vi "Msg Listened To.vi"(7 "Actor in":refnum<class "Actor.lvclass">) -> (2 "Msg Listened To":bool)   [LabVIEW 2020, in "jettl.lvlib"]
uses:
  jettl.lvlib
  Actor/Actor.lvclass
  Msg/Msg.lvclass
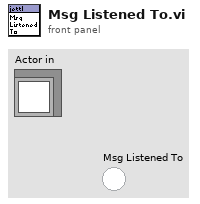
[diagram p1: front panel]
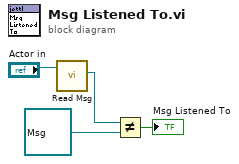
[diagram p0: block diagram]
diagram:
  n1 = call-dynamic "Read Msg.vi"("Actor in"="Actor in") -> ("Msg"=w2:refnum<class "Msg.lvclass">)  [unwired: 10 in]
  n2 = Not Equal?(x=w2, y=refnum<class "Msg.lvclass"> refnum) -> (x != y?=→"Msg Listened To":bool)
